vi "example4.vi"() -> ()   [LabVIEW 2018, in "LV-Julia_ZMQ-Roundtrip_lib.lvlib"]
uses:
  LV-Julia_ZMQ-Roundtrip_lib.lvlib
  Julia functions enum.ctl
  example args cluster.ctl
  example server response cluster.ctl
  Commands v2.ctl
  <vilib>/Analysis/baseanly.llb/Mean (DBL).vi
  <vilib>/Analysis/NI_AALBase.lvlib
panel:
  out "parsed response 2":T1 {"bin_lng" format="%.0e"}
  out "sample size 2":i32
  out "min value 2":dbl
  out "max value 2":dbl
  out "median 2":dbl format="%.6f"
  out "mean 2":dbl format="%.5f"
  in  "fun2call 2":T2=enum."myf3"
  in  "Arguments 2":T3={"arg1"=1, "arg2"=3.14}
  out "roundtrip time 2":dbl
  out "status 2":string
  out "current error 2":errorcluster
  out "parsed response":T1 {"bin_lng" format="%.0e"}
  out "sample size":i32
  in  "bindata size":u32=1
  out "min value":dbl
  out "max value":dbl
  out "median":dbl format="%.6f"
  out "mean":dbl format="%.5f"
  out "final error":errorcluster
  out "current error":errorcluster
  out "status":string
  in  "stop":bool
  out "roundtrip time":dbl
  in  "Arguments":T3={"arg1"=1, "arg2"=3.14}
  in  "fun2call":T2
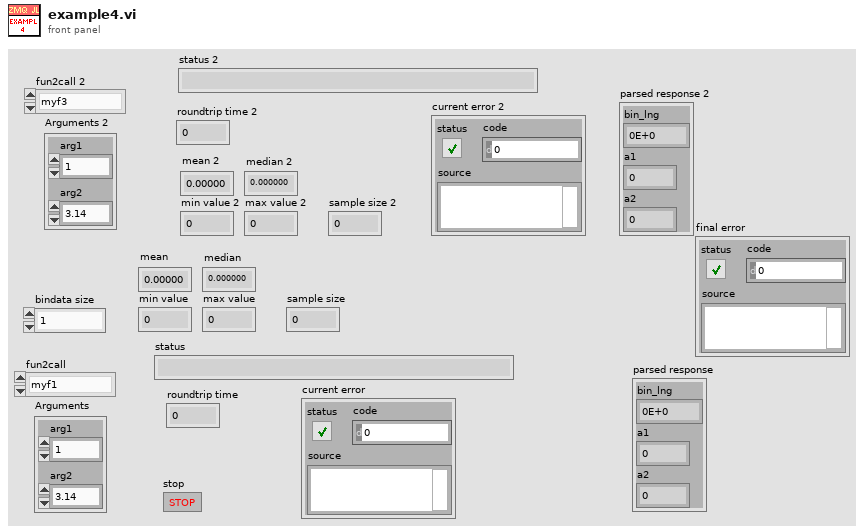
[diagram p1: front panel]
types:
  T1 = typedef "example server response cluster.ctl" = cluster{"bin_lng":i32, "a1":i32, "a2":dbl}
  T2 = typedef "LV-Julia_ZMQ-Roundtrip_lib.lvlib/Julia functions enum.ctl" = enum16{"myf1", "myf2", "myf3", "test_bin2nums", "test_rgbimg", "numarr_loopback", "numarrs_lpbk", "Not_a_Fun"}
  T3 = typedef "example args cluster.ctl" = cluster{"arg1":i32, "arg2":dbl}
  T4 = typedef "LV-Julia_ZMQ-Roundtrip_lib.lvlib/Commands v2.ctl" = enum16{"Start Jl-server & Init LV-client", "Send request & Get response ", "Stop Jl-server & Cleanup LV-client", "Cleanup LV-client", "Start Jl-server", "Stop Jl-server", "Init LV-Client", "Cleanup LV-Client", "(not allowed)", "Set LV Client state", "Set Jl Server state"}
  T5 = typedef "LV-Julia_ZMQ-Roundtrip_lib.lvlib/detailed error info.ctl" = cluster{"exception_or_info":string, "trace":T6[]}
  T6 = typedef "LV-Julia_ZMQ-Roundtrip_lib.lvlib/StackFrame.ctl" = cluster{"frame_summary":string, "func":string, "linfo":string, "file":string, "line":i32, "pointer":u64, "from_c":bool, "inlined":bool}
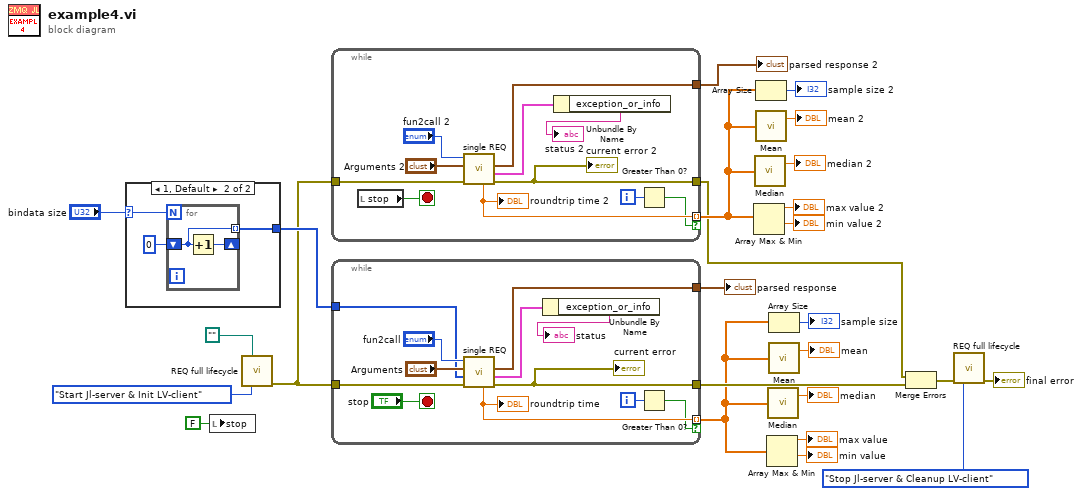
[diagram p0: block diagram]
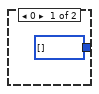
[diagram p2: hidden frame]
diagram:
  n1 = case shown="1, Default" "bindata size" {
    selector: "bindata size" -> [_ w29]
    tunnel: [u8[] [] w27] -> w16
    frame 0 {
    }
    frame 1, Default {
      n2 = for {
        N: w29 -> [_]
        shift-right: [w31] -> _
        shift-left: u8 0 -> [w30]
        tunnel: [w30] -> w27 mode=indexing
        n3 = Increment(x=w30) -> (x+1=w31:u8)
      }
    }
  }
  n4 = local write "stop"(FALSE ("stop")) -> ()
  n5 = call "REQ full lifecycle.vi"("Julia user functions script"=path "", "command"=Commands_v2."Start Jl-server & Init LV-client") -> ("error out"=w5:errorcluster)  [unwired: 10 in, 3 out]
  n6 = while {
    tunnel: w5 -> [w42]
    tunnel: [w41] -> w3
    tunnel: [w38] -> w8 mode=indexing if=w36
    tunnel: [w35] -> w6
    i -> [w37]
    stop <- w34 stop-if-true
    n7 = local read "stop"() -> (w34:bool)
    n8 = call "single REQ.vi"("error in (no error)"=w42, "Arguments"="Arguments 2", "fun2call"="fun2call 2") -> ("error out"=w41:errorcluster, "detailed error info"=w33:T5, "parsed response"=w35:T1, "roundtrip time"=w38:dbl)  [unwired: 3 in, 1 out]
    "roundtrip time 2" <- w38
    "current error 2" <- w41
    n9 = Unbundle By Name(w33) -> ("exception_or_info"=→"status 2":string)
    n10 = Greater Than 0?(x=w37) -> (x > 0?=w36:bool)
  }
  "parsed response 2" <- w6
  n11 = while {
    tunnel: w5 -> [w54]
    tunnel: [w53] -> w25
    tunnel: [w49] -> w15 mode=indexing if=w47
    tunnel: w16 -> [w46]
    tunnel: [w45] -> w13
    i -> [w48]
    stop <- "stop" stop-if-true
    n12 = call "single REQ.vi"("error in (no error)"=w54, "binary data in"=w46, "Arguments"="Arguments", "fun2call"="fun2call") -> ("error out"=w53:errorcluster, "detailed error info"=w44:T5, "parsed response"=w45:T1, "roundtrip time"=w49:dbl)  [unwired: 2 in, 1 out]
    "roundtrip time" <- w49
    "current error" <- w53
    n13 = Unbundle By Name(w44) -> ("exception_or_info"=→"status":string)
    n14 = Greater Than 0?(x=w48) -> (x > 0?=w47:bool)
  }
  "parsed response" <- w13
  n15 = Array Max & Min(array=w8) -> (max value=→"max value 2":dbl, min value=→"min value 2":dbl)  [unwired: 2 out]
  n16 = call <vilib>:"Median.vi"("X"=w8) -> ("median"=→"median 2":dbl)  [unwired: 1 out]
  n17 = Array Size(array=w8) -> (size(s)=→"sample size 2":i32)
  n18 = call-poly <vilib>:"Mean.vi"("X"=w8) -> ("mean"=→"mean 2":dbl)  [unwired: 1 out]
  n19 = Array Max & Min(array=w15) -> (max value=→"max value":dbl, min value=→"min value":dbl)  [unwired: 2 out]
  n20 = call <vilib>:"Median.vi"("X"=w15) -> ("median"=→"median":dbl)  [unwired: 1 out]
  n21 = Array Size(array=w15) -> (size(s)=→"sample size":i32)
  n22 = call-poly <vilib>:"Mean.vi"("X"=w15) -> ("mean"=→"mean":dbl)  [unwired: 1 out]
  n23 = Merge Errors(w3, w25) -> (w4:errorcluster)
  n24 = call "REQ full lifecycle.vi"("error in"=w4, "command"=Commands_v2."Stop Jl-server & Cleanup LV-client") -> ("error out"=→"final error":errorcluster)  [unwired: 10 in, 3 out]
